vi "Set SkipNameAttrAtThisLevel.vi"(8 "error in (no error)":errorcluster, 10 "SkipNameAttrAtThisLevel":bool, 11 "NextGenXMLTypeGenerator.lvclass in":refnum<class "NextGenXMLTypeGenerator.lvclass">) -> (0 "error out":errorcluster, 3 "NextGenXMLTypeGenerator.lvclass out":refnum<class "NextGenXMLTypeGenerator.lvclass">)   [LabVIEW 2020, in "Web Service Description.lvlib" / "NextGenXMLTypeGenerator.lvclass"]
uses:
  <vilib>/AppBuilder/Engine/WebServiceDescription/NextGenXMLTypeGenerator/NextGenXMLTypeGenerator.lvclass
  <vilib>/AppBuilder/Engine/WebServiceDescription/NextGenXMLTypeGenerator/NextGenXMLTypeGenerator.lvclass/NextGenXMLTypeGenerator.ctl
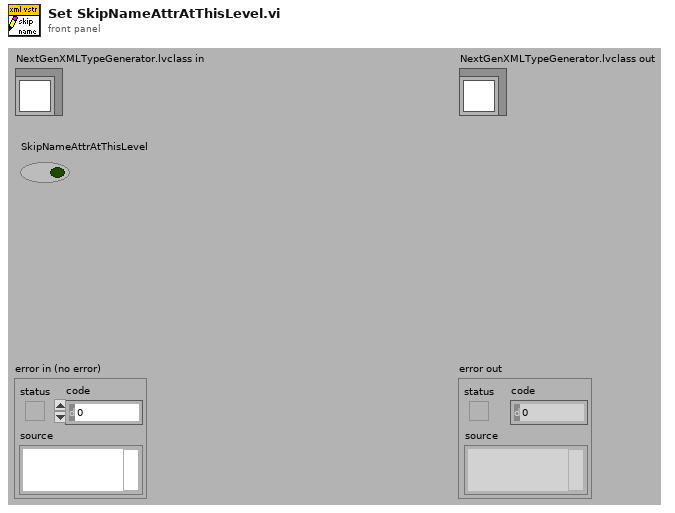
[diagram p1: front panel]
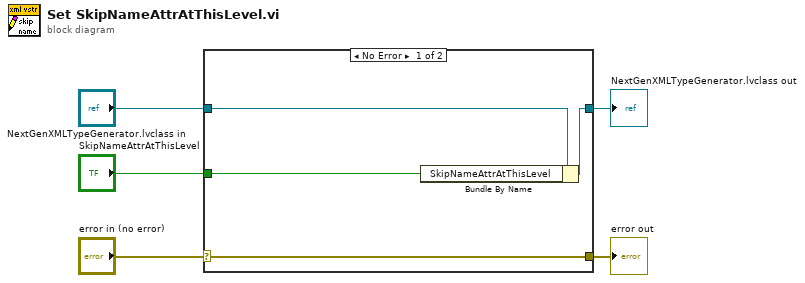
[diagram p0: block diagram]
diagram:
  n1 = case shown="No Error" "error in (no error)" {
    selector: "error in (no error)" -> [w9 w10]
    tunnel: [w9 w10] -> w4
    tunnel: [w7 w11] -> w2
    tunnel: "NextGenXMLTypeGenerator.lvclass in" -> [w8 w11]
    tunnel: "SkipNameAttrAtThisLevel" -> [w6 _]
    frame No Error {
      n2 = Bundle By Name(cluster=w8, "SkipNameAttrAtThisLevel"=w6) -> (w7:refnum<class "NextGenXMLTypeGenerator.lvclass">)
    }
    frame Error {
    }
  }
  "error out" <- w4
  "NextGenXMLTypeGenerator.lvclass out" <- w2
